vi "Move-Axis-Sync.vi"(10 "Speed X":i32, 11 "x mm":dbl) -> ()   [LabVIEW 2017]
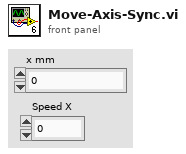
[diagram p1: front panel]
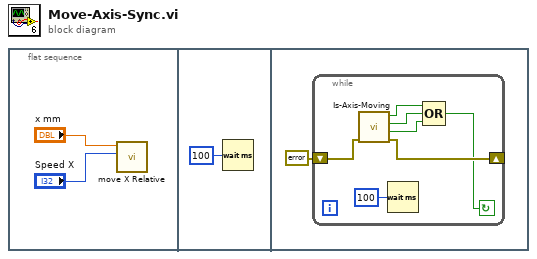
[diagram p0: block diagram]
diagram:
  n1 = flat-sequence {
    frame #0 {
      n2 = call "move X Relative.vi"("Speed X"="Speed X", "x mm"="x mm") -> ()  [unwired: 10 in]
    }
    frame #1 {
      n3 = Wait (ms)(milliseconds to wait=u32 100) -> ()  [unwired: 1 out]
    }
    frame #2 {
      n4 = while {
        shift-right: [w9] -> _
        shift-left: errorcluster {"status"=FALSE, "code"=0, "source"=""} ("error out") -> [w10]
        stop <- w5 continue-if-true
        n5 = call "Is-Axis-Moving.vi"("error in"=w10) -> ("error out"=w9:errorcluster, "Z"=w6:bool, "Y"=w7:bool, "X"=w8:bool)  [unwired: 7 in]
        n6 = Wait (ms)(milliseconds to wait=u32 100) -> ()  [unwired: 1 out]
        n7 = Compound Arithmetic op=OR(w8, w7, w6) -> (w5:bool)
      }
    }
  }
